vi "Check If Keys Unique.vi"(8 "error in (no error)":errorcluster, 11 "Bundle Builder in":refnum<class "Bundle Builder.lvclass">) -> (0 "error out":errorcluster, 1 "Custom Action Key Unique?":bool, 2 "Product Key Unique?":bool, 3 "Bundle Builder out":refnum<class "Bundle Builder.lvclass">)   [LabVIEW 2020, in "Bundle Builder.lvclass"]
uses:
  Bundle Builder.lvclass
  Bundle Builder.lvclass/Bundle Builder.ctl
  27e5509a-78bc-4668-a612-3c7a6fb23583.vi
  296b4c47-4cf8-472a-ba40-33d9fc724dc0.vi
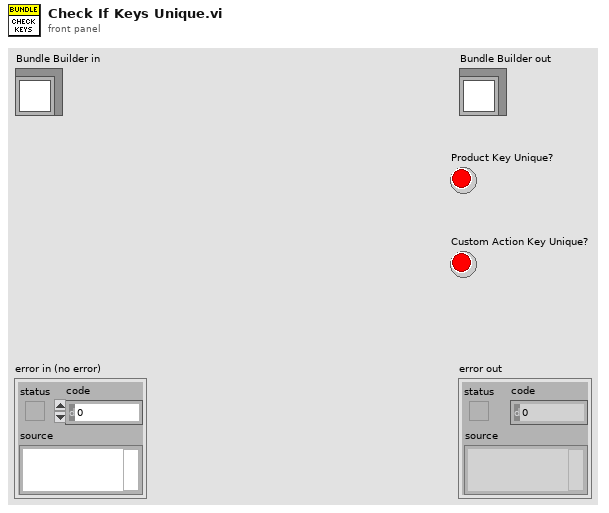
[diagram p1: front panel]
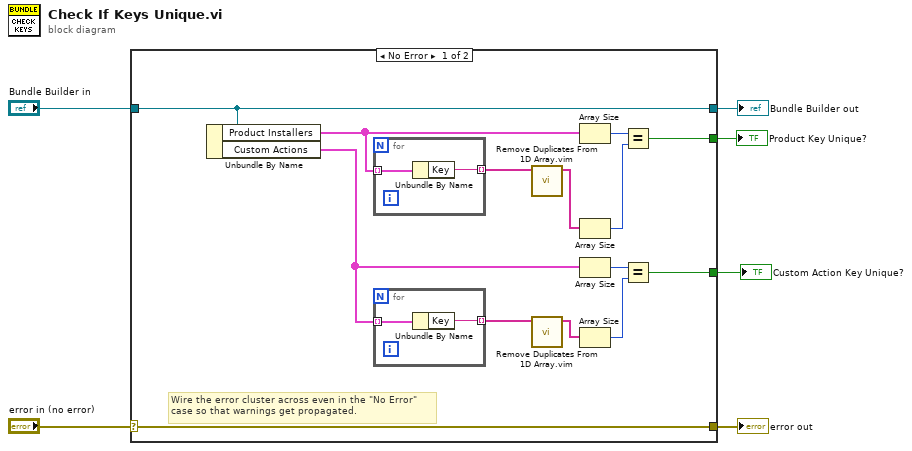
[diagram p0: block diagram]
diagram:
  n1 = case shown="No Error" "error in (no error)" {
    selector: "error in (no error)" -> [w20 w26]
    tunnel: [w20 w26] -> w5
    tunnel: [w19 w25] -> w3
    tunnel: "Bundle Builder in" -> [w19 w25]
    tunnel: [w12 _] -> w2
    tunnel: [w11 _] -> w1
    frame No Error {
      # "Wire the error cluster across even in the \"No Error\"\ncase so that warnings get propagated."
      n2 = Unbundle By Name(w19) -> ("Product Installers"=w10:cluster{"Key":string, "Version":string}[], "Custom Actions"=w8:cluster{"Key":string, "Timing":string}[])
      n3 = for {
        tunnel: w10 -> [w24] mode=indexing
        tunnel: [w23] -> w9 mode=indexing
        n4 = Unbundle By Name(w24) -> ("Key"=w23:string)
      }
      n5 = for {
        tunnel: w8 -> [w22] mode=indexing
        tunnel: [w21] -> w7 mode=indexing
        n6 = Unbundle By Name(w22) -> ("Key"=w21:string)
      }
      n7 = call "Remove Duplicates From 1D Array.vim"("array"=w9) -> ("array with duplicates removed"=w17:string[])  [unwired: 10 in]
      n8 = call "Remove Duplicates From 1D Array.vim"("array"=w7) -> ("array with duplicates removed"=w14:string[])  [unwired: 10 in]
      n9 = Array Size(array=w10) -> (size(s)=w18:i32)
      n10 = Array Size(array=w17) -> (size(s)=w16:i32)
      n11 = Array Size(array=w8) -> (size(s)=w13:i32)
      n12 = Array Size(array=w14) -> (size(s)=w15:i32)
      n13 = Equal?(x=w18, y=w16) -> (x = y?=w11:bool)
      n14 = Equal?(x=w13, y=w15) -> (x = y?=w12:bool)
    }
    frame Error {
    }
  }
  "error out" <- w5
  "Bundle Builder out" <- w3
  "Custom Action Key Unique?" <- w2
  "Product Key Unique?" <- w1
